vi "get hdf dataset shape.vi"(0 "file":string, 1 "ndims":i32, 5 "monitor_id":string, 7 "datasetName":string, 9 "shape":i32) -> (3 "ndims out":i32, 4 "file out":string, 6 "monitor_id out":string, 8 "datasetName out":string, 10 "shape out":i32, 14 "function return":i32)   [LabVIEW 2019, in "apdm.lvlib"]
doc: "APDM_EXPORT int apdm_get_hdf_dataset_shape(char *file, char *monitor_id, char *datasetName, int *shape, int *ndims);"
uses:
  apdm.lvlib
  Lee Lab/CP FES Walking 2018/Code/Working/LabVIEW/apdm.dll
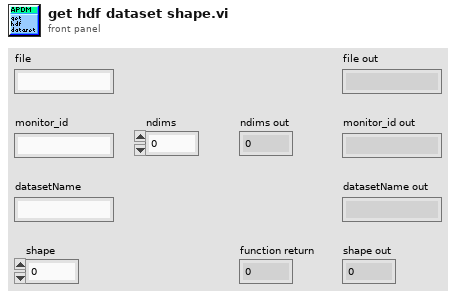
[diagram p1: front panel]
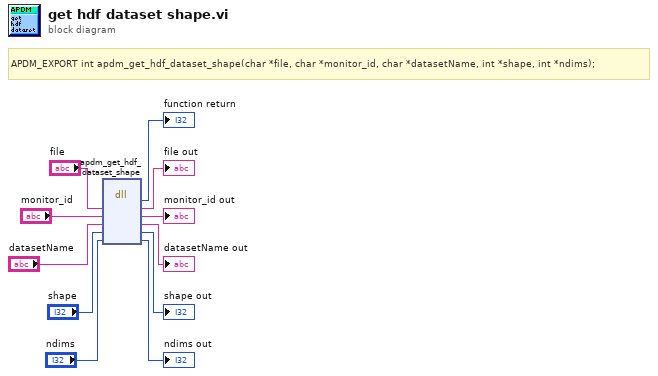
[diagram p0: block diagram]
diagram:
  # "APDM_EXPORT\tint apdm_get_hdf_dataset_shape(char *file, char *monitor_id, char *datasetName, int *shape, int *ndims);"
  n1 = dll-call lib="C:/Users/jfalesi/Dropbox/Lee Lab/CP FES Walking 2018/Code/Working/LabVIEW/apdm.*" fn="apdm_get_hdf_dataset_shape"("file"="file", "monitor_id"="monitor_id", "datasetName"="datasetName", "shape"="shape", "ndims"="ndims") -> (→"function return":i32, "file"=→"file out":string, "monitor_id"=→"monitor_id out":string, "datasetName"=→"datasetName out":string, "shape"=→"shape out":i32, "ndims"=→"ndims out":i32)  [unwired: 3 in, 2 out]
